vi "Sample Image.vi"() -> (3 "Sample Image image/TIFF":string)   [LabVIEW 2014]
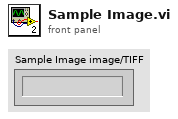
[diagram p1: front panel]
diagram:
  "Sample Image image/TIFF" <- "II*\u0000D%\u0000à/À0ð0@,01@.p2\u00002 2/\u00004 2À0 1 1\u0000+\u00105P4à2à+\u00100P.P6@1à0à-,@0 /5000: 5`303\u00108 5`/p1 3à/à9 3Ð2\u0010.ð0P/ 2\u00000 3 3à/`. : 2à,02à2`;à-ð1@3p20506À-Ð,À2\u00005`-@/à20.`1à(p+01à20 5 / 2`.à/ 0+08,ð8à%+P0 (à2+ 7 5) +à1P)à+ .à1 1Ð1à. 2à.@+0)ð.\u0000.À)°22à.À. 2 / 0 0`/Ð0 +0*Ð/À,°5\u00008 -`3 0 2p3 0 0 1`-\u0000,\u00101@,\u00105ð. .p*à,6 .à0#à4°&°.P%À+`-À/p)`9°2/@-àR`.P0 2\u00003°1À/ / . 00>\u00105Ð* $à+ /+°)p(À(`0 1`/°0°'0-Ð'.`*/0/ ,à2 1*@/P+ð)Ð, *0.( 1ð(\u00100`+ 0°Và8\u0010(p+p)`# $P(Ð(0-p( )@#P+à'P-0'à+%à+Ð, ).°- ! %`0\u0000+\u0000*0* %@- (\u0000,À.@-P*p' * *+*Ð3\u0010)°)ð0À+ +(à*à. ' &ð. -à-°/à*P' 2ð,* *`(Ð-`$p4 ' + /0\"ð,\u0010*à*p%`2 ' ' + 0à,@)°&`,,*..." ("body 2")
